vi "Write_from_Sensor.vi"() -> ()   [LabVIEW 2018]
uses:
  <vilib>/measure/NI_MABase.lvlib
panel:
  out "웨이브폼 차트":waveform(dbl)(graph)
  out "signal out":waveform(dbl) caption="신호 출력"
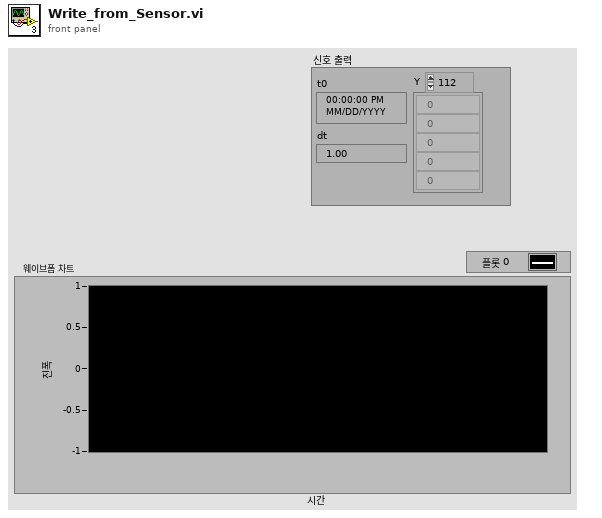
[diagram p1: front panel]
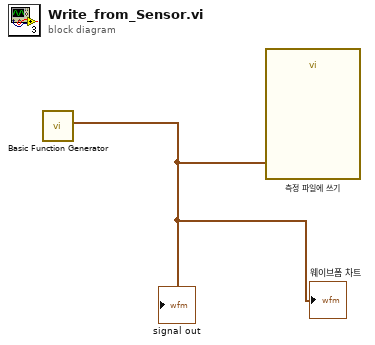
[diagram p0: block diagram]
diagram:
  n1 = call <vilib>:"Basic Function Generator.vi"() -> ("signal out"=w1:waveform(dbl))  [unwired: 9 in, 2 out]
  "signal out" <- w1
  "웨이브폼 차트" <- w1
  n2 = call "측정 파일에 쓰기"("Signals"=w1) -> ()  [unwired: 16 in, 3 out]
